vi "Configure.vi"(6 "Series CFG":string, 8 "error in":errorcluster, 9 "Virt Instrs":string, 10 "Instr CFGs":string[](array[string]), 11 "Series Actor in":refnum<class "Series Actor.lvclass">) -> (0 "error out":errorcluster, 3 "Series Actor out":refnum<class "Series Actor.lvclass">)   [LabVIEW 2023, in "Series Actor.lvlib" / "Series Actor.lvclass"]
uses:
  Series Actor.lvclass
  Series Actor.lvclass/Series Actor.ctl
  <vilib>/JDP Science/JSONtext/Next JSON Value.vi
  <vilib>/JDP Science/JSONtext/String Subset.vi
  <vilib>/JDP Science/JSONtext/Parsing/Advance past next JSON Value (inlined COPY).vi
  <vilib>/JDP Science/JSONtext/Parsing/Advance past whitespace.vi
  <vilib>/JDP Science/JSONtext/Parsing/Advance past String.vi
  <vilib>/JDP Science/JSONtext/Parsing/Advance past Number.vi
  <vilib>/JDP Science/JSONtext/Parsing/Advance past Line Ending.vi
  <vilib>/Utility/error.llb/Error Cluster From Error Code.vi
  <vilib>/JDP Science/JSONtext/Parsing/Parse Full Path or Item Name.vi
  <vilib>/JDP Science/JSONtext/Parsing/Advance past Array.vi
  <vilib>/JDP Science/JSONtext/Parsing/Advance past Object.vi
  <vilib>/JDP Science/JSONtext/support/Error Cluster From Code.vi
  <vilib>/JDP Science/JSONtext/Offset/Find Item Locations by Path.vi
  <vilib>/JDP Science/JSONtext/support/Format JSON Array Text.vi
  <vilib>/ErrorRing/Error Ring.xnode
  <vilib>/JDP Science/JSONtext/JSONtext.lvlib
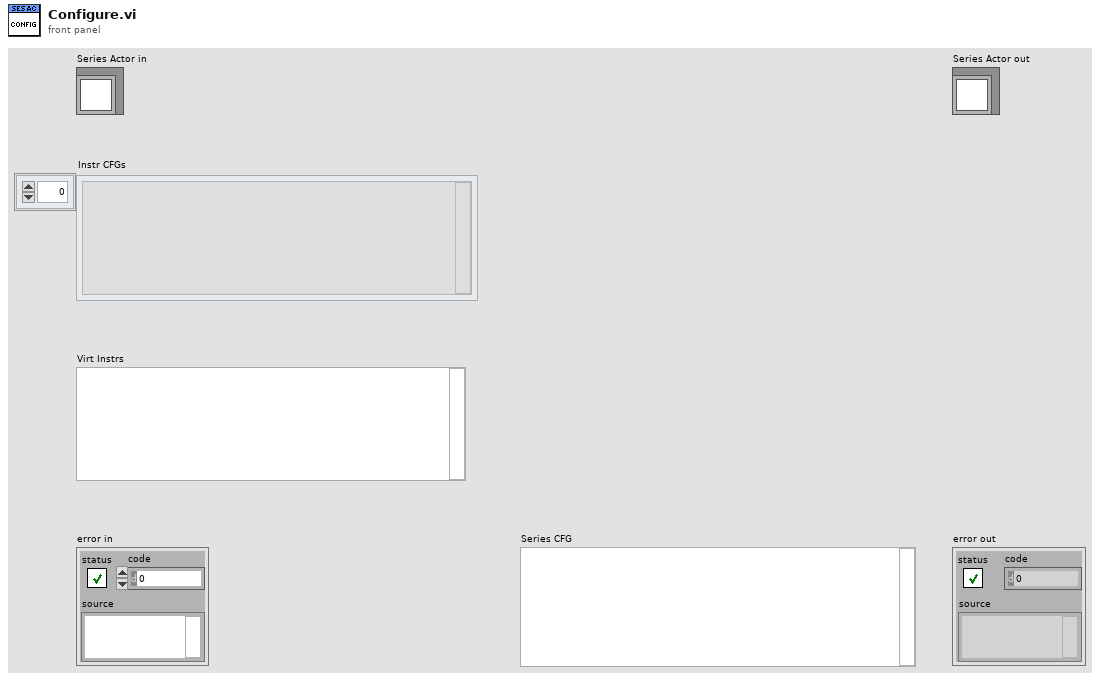
[diagram p1: front panel]
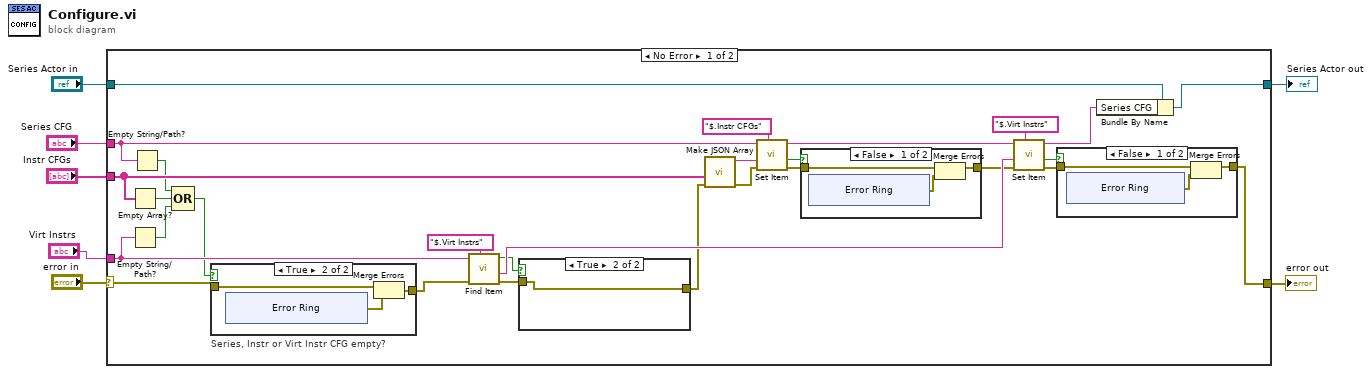
[diagram p0: block diagram]
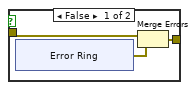
[diagram p5: hidden frame]
diagram:
  n1 = case shown="No Error" "error in" {
    selector: "error in" -> [w13 w72]
    tunnel: [w17 w72] -> w4
    tunnel: [w34 w73] -> w6
    tunnel: "Series Actor in" -> [w35 w73]
    tunnel: "Virt Instrs" -> [w15 _]
    tunnel: "Series CFG" -> [w14 _]
    tunnel: "Instr CFGs" -> [w16 _]
    frame No Error {
      n2 = Empty Array?(array=w16) -> (empty?=w11:bool)
      n3 = Empty String/Path?(string/path=w15) -> (empty?=w10:bool)
      n4 = Empty String/Path?(string/path=w14) -> (empty?=w12:bool)
      n5 = Compound Arithmetic op=OR(w12, w11, w10) -> (w9:bool)
      n6 = case "Series, Instr or Virt Instr CFG empty?" shown="True" w9 {
        tunnel: w13 -> [w36 w39]
        tunnel: [w36 w38] -> w8
        frame False {
        }
        frame True {
          n7 = xnode "Error Ring"() -> ("error out"=w37:errorcluster)
          n8 = Merge Errors(w39, w37) -> (w38:errorcluster)
        }
      }
      n9 = call <vilib>:"Find Item.vi"("$Path or Item Name"="$.Virt Instrs", "error in (no error)"=w8, "JSON"=w15) -> ("error out"=w23:errorcluster, "<JSON>"=w25:string, "Found"=w24:bool)  [unwired: 5 in, 1 out]
      n10 = case shown="True" w24 {
        tunnel: w23 -> [w65 w71]
        tunnel: [w63 w71] -> w22
        frame False {
          n11 = xnode "Error Ring"() -> ("error out"=w64:errorcluster)
          n12 = Merge Errors(w65, w64) -> (w63:errorcluster)
        }
        frame True {
        }
      }
      n13 = call <vilib>:"Make JSON Array.vi"("error in (no error)"=w22, "JSON Elements"=w16) -> ("error out"=w29:errorcluster, "<JSON>"=w31:string)  [unwired: 8 in]
      n14 = call <vilib>:"Set Item.vi"("$Path or Item Name"="$.Instr CFGs", "error in (no error)"=w29, "JSON to Insert"=w31, "JSON"=w14) -> ("error out"=w28:errorcluster, "Replaced"=w20:bool, "<JSON>"=w27:string)  [unwired: 4 in]
      n15 = case shown="False" w20 {
        tunnel: w28 -> [w56 w62]
        tunnel: [w55 w62] -> w21
        frame False {
          n16 = xnode "Error Ring"() -> ("error out"=w54:errorcluster)
          n17 = Merge Errors(w56, w54) -> (w55:errorcluster)
        }
        frame True {
        }
      }
      n18 = call <vilib>:"Set Item.vi"("$Path or Item Name"="$.Virt Instrs", "error in (no error)"=w21, "JSON to Insert"=w25, "JSON"=w27) -> ("error out"=w18:errorcluster, "Replaced"=w19:bool, "<JSON>"=w32:string)  [unwired: 4 in]
      n19 = case shown="False" w19 {
        tunnel: w18 -> [w47 w53]
        tunnel: [w46 w53] -> w17
        frame False {
          n20 = xnode "Error Ring"() -> ("error out"=w45:errorcluster)
          n21 = Merge Errors(w47, w45) -> (w46:errorcluster)
        }
        frame True {
        }
      }
      n22 = Bundle By Name(cluster=w35, "Series CFG"=w32) -> (w34:refnum<class "Series Actor.lvclass">)
    }
    frame Error {
    }
  }
  "error out" <- w4
  "Series Actor out" <- w6
